vi "VariableWrite.vi"(8 "error in (no error)":errorcluster, 9 "OriginalName":string, 10 "Variable":refnum<class "Variable.lvclass">, 11 "VariablesManager in":refnum<class "VariableManager.lvclass">) -> (0 "error out":errorcluster, 3 "VariablesManager out":refnum<class "VariableManager.lvclass">)   [LabVIEW 2013, in "VariableManager.lvclass"]
doc: "Add the given variable definition to database.\nTo overwrite existing variable definition, provide the OriginalName.\n\nAn error is thrown if the given Variable is malformed, failing the test in VariableCheck.vi"
uses:
  VariableManager.lvclass
  Variable/Variable.lvclass
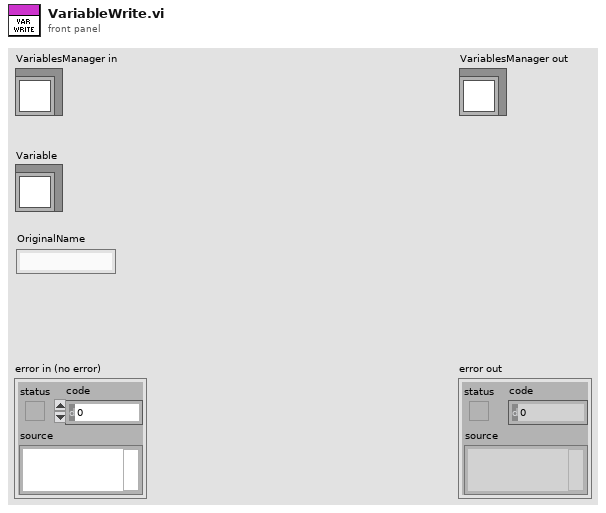
[diagram p1: front panel]
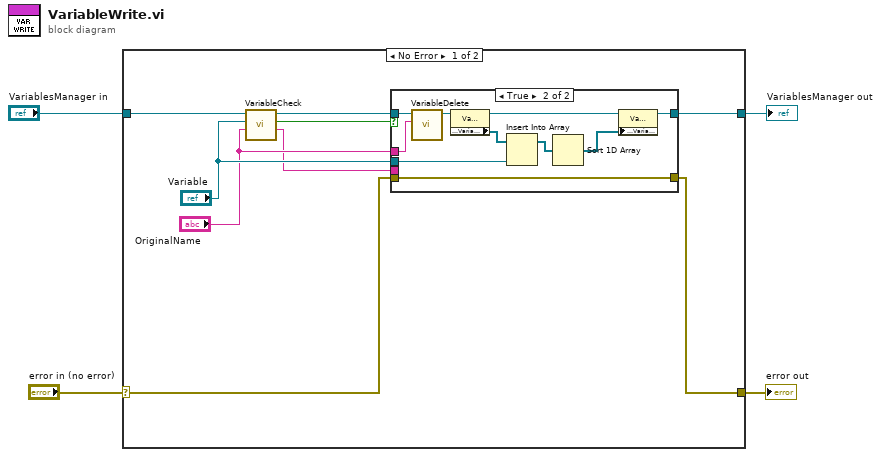
[diagram p0: block diagram]
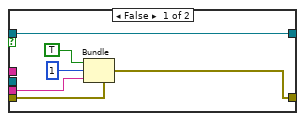
[diagram p2: hidden frame]
diagram:
  n1 = case shown="No Error" "error in (no error)" {
    selector: "error in (no error)" -> [w7 w31]
    tunnel: [w5 w31] -> w3
    tunnel: [w13 w30] -> w1
    tunnel: "VariablesManager in" -> [w12 w30]
    frame No Error {
      n2 = call-dynamic "VariableCheck.vi"("OriginalName"="OriginalName", "VariableIn"="Variable", "VariableManager in"=w12) -> ("RejectMessage"=w6:string, "Pass"=w10:bool, "VariableManager out"=w11:refnum<class "VariableManager.lvclass">)  [unwired: 5 in, 1 out]
      n3 = case shown="True" w10 {
        tunnel: [w19 w25] -> w13
        tunnel: w11 -> [w19 w23]
        tunnel: "Variable" -> [_ w22]
        tunnel: "OriginalName" -> [_ w21]
        tunnel: w7 -> [w18 w20]
        tunnel: w6 -> [w15 _]
        tunnel: [w14 w20] -> w5
        frame False {
          n4 = Bundle(cluster=w18, "status"=TRUE, "code"=1, "source"=w15) -> (w14:errorcluster)
        }
        frame True {
          n5 = call-dynamic "VariableDelete.vi"("VariableName"=w21, "VariablesManager in"=w23) -> ("VariablesManager out"=w24:refnum<class "VariableManager.lvclass">)  [unwired: 8 in, 1 out]
          n6 = property class="VariableManager.lvclass"(reference=w24) -> (reference out=w29:refnum<class "VariableManager.lvclass">, "Accessors:Variables"=w28:refnum<class "Variable.lvclass">[])  [unwired: 1 in, 1 out]
          n7 = Insert Into Array(array=w28, new element=w22) -> (w27:refnum<class "Variable.lvclass">[])  [unwired: 1 in]
          n8 = Sort 1D Array(array=w27) -> (sorted array=w26:refnum<class "Variable.lvclass">[])
          n9 = property class="VariableManager.lvclass"(reference=w29, "Accessors:Variables"=w26) -> (reference out=w25:refnum<class "VariableManager.lvclass">)  [unwired: 1 in, 1 out]
        }
      }
    }
    frame Error {
    }
  }
  "error out" <- w3
  "VariablesManager out" <- w1
